vi "Empty LUT.vi"(8 "error in (no error)":errorcluster, 11 "LUT in":refnum<class "LUT.lvclass">) -> (0 "error out":errorcluster, 3 "LUT out":refnum<class "LUT.lvclass">)   [LabVIEW 2017, in "LUT.lvlib" / "LUT.lvclass"]
doc: "Deletes all the attributes and associated values."
uses:
  LUT.lvclass
  LUT.lvclass/LUT.ctl
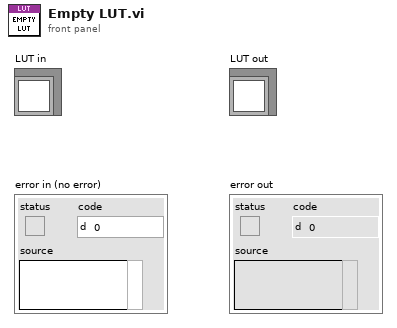
[diagram p1: front panel]
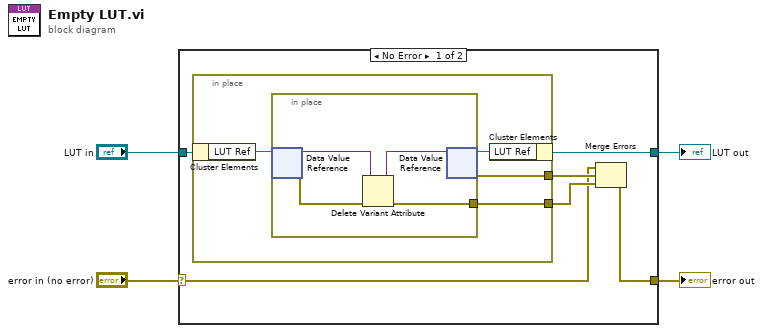
[diagram p0: block diagram]
diagram:
  n1 = case shown="No Error" "error in (no error)" {
    selector: "error in (no error)" -> [w6 w20]
    tunnel: [w5 w20] -> w3
    tunnel: [w9 w19] -> w1
    tunnel: "LUT in" -> [w10 w19]
    frame No Error {
      n2 = in-place {
        in-place-border: [w12] -> w7
        in-place-border: [w11] -> w8
        n3 = in-place-cluster #1(w10) -> ("LUT Ref"=w14:refnum<data-value>)
        n4 = in-place {
          in-place-border: [w16] -> w12
          n5 = in-place-dvr #2(w14) -> (w18:variant, w17:errorcluster)
          n6 = Delete Variant Attribute(4:w17, 7:w18) -> (0:w16:errorcluster, 3:w15:variant)  [unwired: 1 in, 1 out]
          n7 = in-place-dvr #2(w15) -> (w13:refnum<data-value>, w11:errorcluster)
        }
        n8 = in-place-cluster #1("LUT Ref"=w13) -> (w9:refnum<class "LUT.lvclass">)
      }
      n9 = Merge Errors(w6, w8, w7) -> (w5:errorcluster)
    }
    frame Error {
    }
  }
  "error out" <- w3
  "LUT out" <- w1
